vi "Init Msg.vi"(9 "Name Specs":refnum<class "Name Specs.lvclass">, 10 "Project Stuff":refnum<class "Project Stuff.lvclass">) -> (3 "Msg out":refnum<class "Msg.lvclass">)   [LabVIEW 2020, in "_Rescript.lvlib" / "Msg.lvlib" / "Msg.lvclass"]
uses:
  Msg.lvclass
  _Shared/Project Stuff/Project Stuff.lvclass
  _Shared/Name Specs/Name Specs.lvclass
  Msg.lvclass/Msg.ctl
  Terminals.ctl
  _Rescript.lvlib
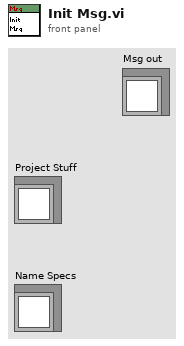
[diagram p1: front panel]
types:
  T1 = typedef "_Rescript.lvlib/Terminals.ctl" = set{i32}
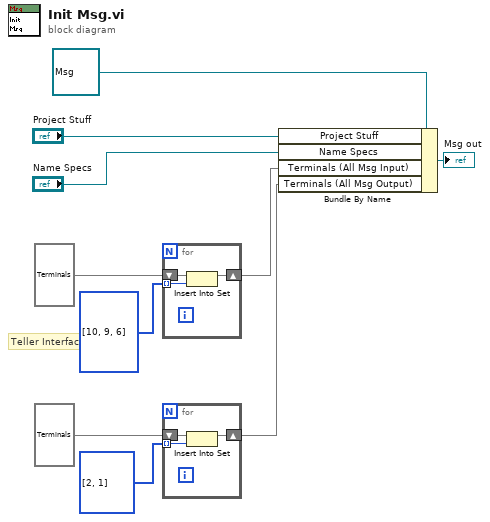
[diagram p0: block diagram]
diagram:
  # "Teller Interface (6)"
  n1 = for {
    tunnel: i32[] [10, 9, 6] -> [w11] mode=indexing
    shift-right: [w12] -> w2
    shift-left: T1 {} ("All Terminals") -> [w13]
    n2 = Insert Into Set(10:w11, 11:w13) -> (3:w12:T1)  [unwired: 1 out]
  }
  n3 = for {
    tunnel: i32[] [2, 1] -> [w14] mode=indexing
    shift-right: [w15] -> w1
    shift-left: T1 {} ("All Terminals") -> [w16]
    n4 = Insert Into Set(10:w14, 11:w16) -> (3:w15:T1)  [unwired: 1 out]
  }
  n5 = Bundle By Name(cluster=refnum<class "Msg.lvclass"> refnum ("Msg out"), "Project Stuff"="Project Stuff", "Name Specs"="Name Specs", "Terminals (All Msg Input)"=w2, "Terminals (All Msg Output)"=w1) -> (→"Msg out":refnum<class "Msg.lvclass">)
